vi "Fit to Square Pulse.vi"(6 "Square Pulse Options":T4={"Method"=enum."Mode", "# Bins"=0, "Threshold %"=10.0, "Center on Midpoint"=TRUE, "Smoothen Plot"=FALSE}, 8 "error in (no error)":errorcluster, 11 "Selected Plot Info":T1={"Multiplot XY Graph"=refnum, "Mouse Coordinates"={"Horizontal"=0, "Vertical"=0}, "Plot Index"=-1}) -> (0 "Error Out":errorcluster, 1 "Fitted Plot Message":string, 3 "Fitted Plot":T6)   [LabVIEW 2021, in "Fits.lvlib"]
uses:
  Square Pulse Options.ctl
  Square Pulse Levels Type.ctl
  Graphs/XY Graph/XY Graph Selected Plot Info.ctl
  Graphs/XY Graph/XY Graph Refnum.ctl
  <vilib>/Utility/miscctls.llb/LVPoint32TypeDef.ctl
  Graphs/XY Graph/XY Graph Add Single Plot with Name.vi
  Fits.lvlib
  Graphs/XY Graph/XY Graph Add-Ons.lvlib
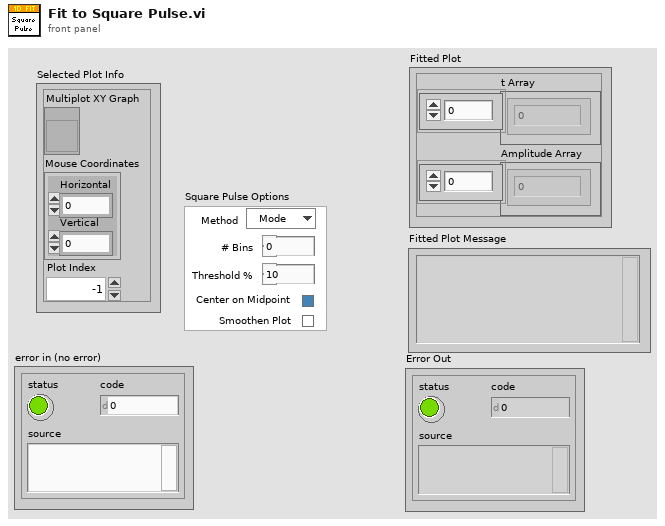
[diagram p1: front panel]
types:
  T1 = typedef "XY Graph Add-Ons.lvlib/XY Graph Selected Plot Info.ctl" = cluster{"Multiplot XY Graph":T2, "Mouse Coordinates":T3, "Plot Index":i32}
  T2 = typedef "XY Graph Add-Ons.lvlib/XY Graph Refnum.ctl" = refnum<vi>
  T3 = typedef "LVPoint32TypeDef.ctl" = cluster{"Horizontal":i32, "Vertical":i32}
  T4 = typedef "Fits.lvlib/Square Pulse Options.ctl" = cluster{"Method":T5, "# Bins":i32, "Threshold %":dbl, "Center on Midpoint":bool, "Smoothen Plot":bool}
  T5 = typedef "Fits.lvlib/Square Pulse Levels Type.ctl" = enum16{"Mode", "Mean"}
  T6 = cluster{"t Array":dbl[], "Amplitude Array":dbl[]}
  T7 = typedef "XY Graph Add-Ons.lvlib/XY Plot Data.ctl" = cluster{"X Array":dbl[], "Y Array":dbl[]}
  T8 = typedef "Fits.lvlib/Square Pulse Statistics.ctl" = cluster{"High Level":dbl, "Low Level":dbl, "Rising Edge Midpoint":dbl, "Falling Edge Midpoint":dbl, "Rising Edge Width":dbl, "Falling Edge Width":dbl}
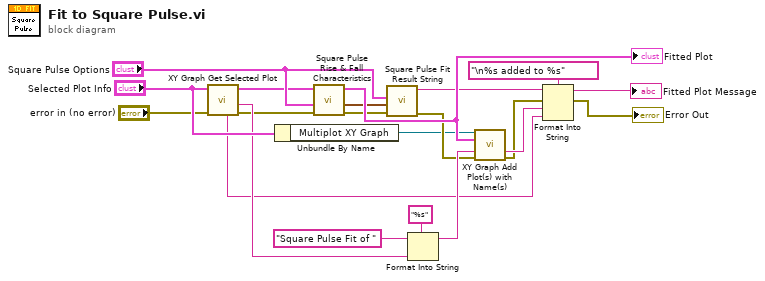
[diagram p0: block diagram]
diagram:
  n1 = call "XY Graph Get Selected Plot.vi"("error in (no error)"="error in (no error)", "Selected Plot Info"="Selected Plot Info") -> ("error out"=w2:errorcluster, "Plot Name"=w4:string, "Plot"=w5:T7, "Graph Name"=w1:string)  [unwired: 4 in, 2 out]
  n2 = Unbundle By Name("Selected Plot Info") -> ("Multiplot XY Graph"=w3:T2)
  n3 = call "Square Pulse Rise & Fall Characteristics.vi"("error in (no error)"=w2, "Square Pulse Options"="Square Pulse Options", "Decay"=w5) -> ("error out"=w12:errorcluster, "Square Pulse Statistics"=w9:T8, "Fitted Decay"=w19:cluster{"t Array":dbl[], "Fitted Array":dbl[]})  [unwired: 4 in, 2 out]
  "Fitted Plot" <- w19
  n4 = call "Square Pulse Fit Result String.vi"("error in (no error)"=w12, "Square Pulse Statistics"=w9, "Square Pulse Options"="Square Pulse Options") -> ("error out"=w11:errorcluster, "Result String"=w10:string)  [unwired: 7 in]
  n5 = Format Into String(format string="%s", initial string="Square Pulse Fit of ", w4) -> (resulting string=w16:string)  [unwired: 1 in, 1 out]
  n6 = call-poly "XY Graph Add Plot(s) with Name(s).vi"("XYGraph Ref in"=w3, "Plot"=w19, "Plot Name (\"Plot\")"=w16, "error in (no error)"=w11) -> ("Plot Name"=w14:string, "error out"=w13:errorcluster)  [unwired: 8 in, 2 out]
  n7 = Format Into String(format string="\n%s added to %s", initial string=w10, error in=w13, w14, w1) -> (resulting string=→"Fitted Plot Message":string, error out=→"Error Out":errorcluster)
